vi ".NET Array Datatype Information to G Array Type Information.vi"(8 "error in (no error)":errorcluster, 9 ".NET Data Type Information":refnum<k24>, 11 "TwinCAT ADS in":refnum<class "TwinCAT ADS.lvclass">) -> (0 "error out":errorcluster, 2 "Array Datatype Information":T1 {"Category" items=["Unknown, None"=0, "Primitive"=1, "Alias"=2, "Enum"=3, "Array"=4, "Struct"=5, "FunctionBlock"=6, "Program"=7, "Function"=8, "SubRange"=9, "String"=10, "Bitset"=12, "Pointer"=13, "Union"=14, "Reference"=15, "Interface"=16]; "Type ID" items=["ADST_VOID"=0, "ADST_INT16"=2, "ADST_INT32"=3, "ADST_REAL32"=4, "ADST_REAL64"=5, "ADST_INT8"=16, "ADST_UINT8"=17, "ADST_UINT16"=18, "ADST_UINT32"=19, "ADST_INT64"=20, "ADST_UINT64"=21, "ADST_STRING"=30, "ADST_WSTRING"=31, "ADST_REAL80"=32, "ADST_BIT"=33, "ADST_MAXTYPES"=34, "ADST_BIGTYPE"=65]}, 3 "TwinCAT ADS out":refnum<class "TwinCAT ADS.lvclass">)   [LabVIEW 2018, in "TwinCAT ADS.lvclass"]
uses:
  TwinCAT ADS.lvclass
  TwinCAT.Ads
  Controls/Array Datatype Information.ctl
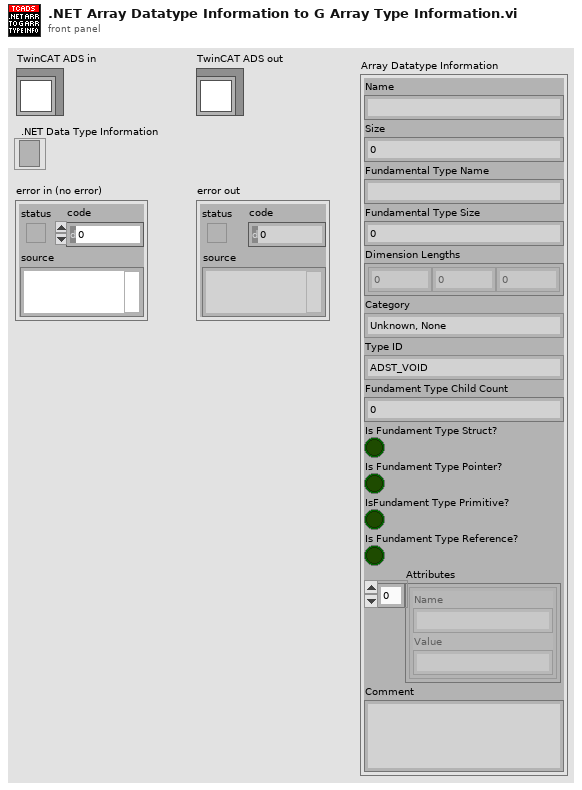
[diagram p1: front panel]
types:
  T1 = typedef "TwinCAT ADS.lvclass/Array Datatype Information.ctl" = cluster{"Name":string, "Size":i32, "Fundamental Type Name":string, "Fundamental Type Size":i32, "Dimension Lengths":i32[], "Category":i32, "Type ID":i32, "Fundament Type Child Count":i32, "Is Fundament Type Struct?":bool, "Is Fundament Type Pointer?":bool, "IsFundament Type Primitive?":bool, "Is Fundament Type Reference?":bool, "Attributes":cluster{"Name":string, "Value":string}[], "Comment":string}
  T2 = typedef "TwinCAT ADS.lvclass/Datatype Information.ctl" = cluster{"Name":string, "Size":i32, "Category":i32, "Type ID":i32, "Child Count":i32, "Is Array?":bool, "Is Struct?":bool, "Is Pointer?":bool, "Is Primitive?":bool, "Is Reference?":bool, "Attributes":cluster{"Name":string, "Value":string}[], "Comment":string}
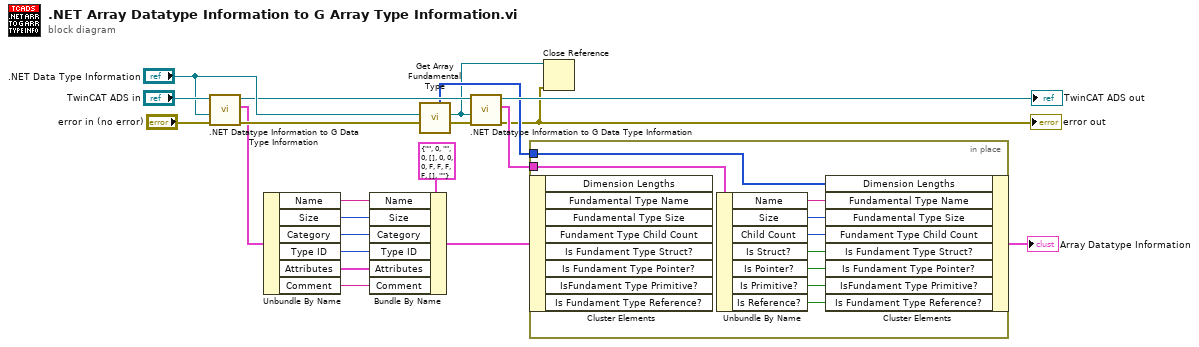
[diagram p0: block diagram]
diagram:
  n1 = call ".NET Datatype Information to G Data Type Information.vi"("error in (no error)"="error in (no error)", ".NET Data Type Information"=".NET Data Type Information", "TwinCAT ADS in"="TwinCAT ADS in") -> ("error out"=w19:errorcluster, "Data Type Information"=w16:T2, "TwinCAT ADS out"=w7:refnum<class "TwinCAT ADS.lvclass">)  [unwired: 6 in]
  n2 = Unbundle By Name(w16) -> ("Name"=w10:string, "Size"=w11:i32, "Category"=w12:i32, "Type ID"=w13:i32, "Attributes"=w14:cluster{"Name":string, "Value":string}[], "Comment"=w15:string)
  n3 = Bundle By Name(cluster=T1 {"Name"="", "Size"=0, "Fundamental Type Name"="", "Fundamental Type Size"=0, "Dimension Lengths"=[], "Category"=0, "Type ID"=0, "Fundament Type Child Count"=0, "Is Fundament Type Struct?"=FALSE, "Is Fundament Type Pointer?"=FALSE, "IsFundament Type Primitive?"=FALSE, "Is Fundament Type Reference?"=FALSE, "Attributes"=[], "Comment"=""} ("Array Datatype Information"), "Name"=w10, "Size"=w11, "Category"=w12, "Type ID"=w13, "Attributes"=w14, "Comment"=w15) -> (w9:T1)
  n4 = call "Get Array Fundamental Type.vi"("error in (no error)"=w19, ".NET AdsDataType"=".NET Data Type Information") -> ("error out"=w8:errorcluster, "Fundametal .NET AdsDataType"=w1:refnum<k24>, "Dimension Lengths"=w4:i32[])  [unwired: 6 in, 1 out]
  n5 = call ".NET Datatype Information to G Data Type Information.vi"("error in (no error)"=w8, ".NET Data Type Information"=w1, "TwinCAT ADS in"=w7) -> ("error out"=w2:errorcluster, "Data Type Information"=w5:T2, "TwinCAT ADS out"=→"TwinCAT ADS out":refnum<class "TwinCAT ADS.lvclass">)  [unwired: 6 in]
  "error out" <- w2
  n6 = in-place {
    in-place-border: w5 -> [w30]
    in-place-border: w4 -> [w29]
    n7 = in-place-cluster #1(w9) -> ()  [unwired: 8 out]
    n8 = Unbundle By Name(w30) -> ("Name"=w28:string, "Size"=w27:i32, "Child Count"=w26:i32, "Is Struct?"=w22:bool, "Is Pointer?"=w23:bool, "Is Primitive?"=w24:bool, "Is Reference?"=w25:bool)
    n9 = in-place-cluster #1("Dimension Lengths"=w29, "Fundamental Type Name"=w28, "Fundamental Type Size"=w27, "Fundament Type Child Count"=w26, "Is Fundament Type Struct?"=w22, "Is Fundament Type Pointer?"=w23, "IsFundament Type Primitive?"=w24, "Is Fundament Type Reference?"=w25) -> (→"Array Datatype Information":T1)
  }
  n10 = Close Reference(reference=w1, error in (no error)=w2) -> ()  [unwired: 1 out]
